vi "19_Sine wave using while loop.vi"() -> ()   [LabVIEW 2018]
panel:
  in  "stop 2":bool
  out "Waveform Graph":dbl[](graph)
  out "Waveform Chart":dbl(graph)
  in  "stop":bool
  # "Develop a HMI to plot sine wave using while loop and display on the waveform graph"
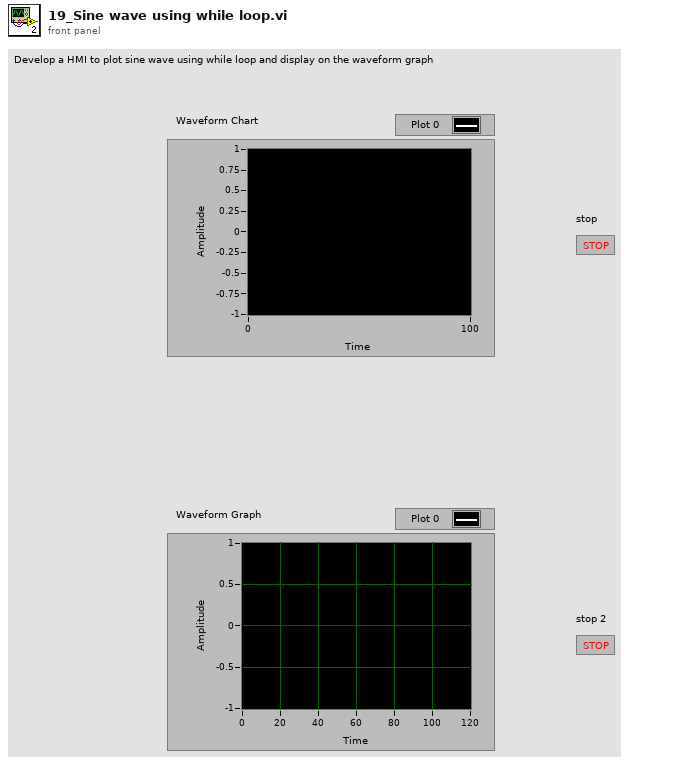
[diagram p1: front panel]
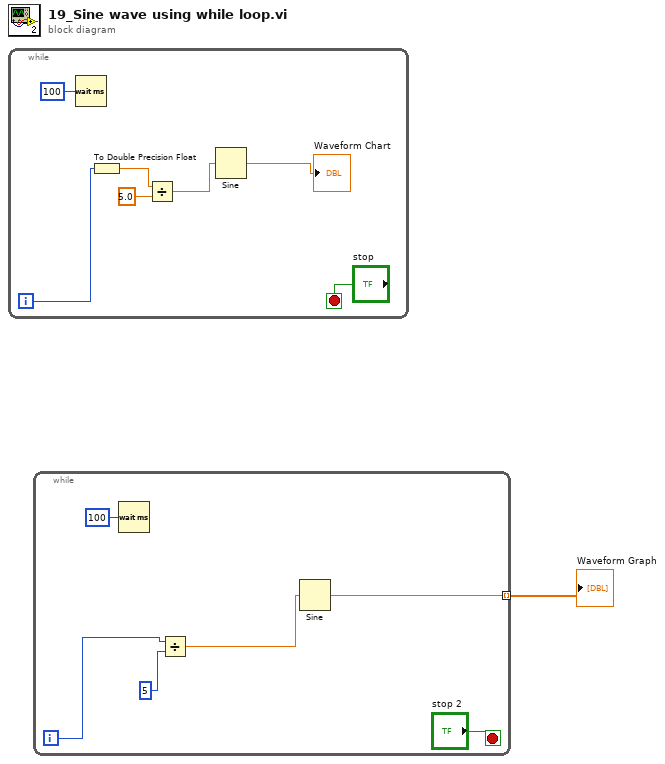
[diagram p0: block diagram]
diagram:
  n1 = while {
    i -> [w5]
    stop <- "stop" stop-if-true
    n2 = Wait (ms)(milliseconds to wait=u32 100) -> ()  [unwired: 1 out]
    n3 = To Double Precision Float(number=w5) -> (double precision float=w4:dbl)
    n4 = Divide(x=w4, y=5.0) -> (x/y=w7:dbl)
    n5 = Sine(x=w7) -> (sin(x)=→"Waveform Chart":dbl)
  }
  n6 = while {
    tunnel: [w11] -> w1 mode=indexing
    i -> [w14]
    stop <- "stop 2" stop-if-true
    n7 = Wait (ms)(milliseconds to wait=u32 100) -> ()  [unwired: 1 out]
    n8 = Divide(x=w14, y=5) -> (x/y=w12:dbl)
    n9 = Sine(x=w12) -> (sin(x)=w11:dbl)
  }
  "Waveform Graph" <- w1
